vi "ValueSignal [Poly].vi"   [LabVIEW 2016]
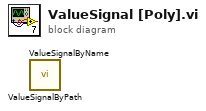
[diagram p0: block diagram]
diagram:
  n1 = call "ValueSignalByPath.vi"() -> ()  [unwired: 14 in, 2 out]
  n2 = call "ValueSignalByName.vi"() -> ()  [unwired: 14 in, 2 out]
